vi "Initialization VI.vi"(8 "error in (no error)":errorcluster, 10 "Custom XML":string, 11 "Device Item Ref in":T1 format="%.0x") -> (0 "error out":errorcluster, 3 "Device Item Ref out":T1 format="%.0x")   [LabVIEW 2019, in "FPGA Addon System Explorer.lvlib"]
uses:
  FPGA Addon System Explorer.lvlib
  <vilib>/NI/NI VeriStand Custom Device Import and Export Tool/ImportExport.lvlib
  Addon Shared/FPGA Addon Shared.lvlib
  <vilib>/NI VeriStand/Custom Device API/Custom Device Item Ref.ctl
  <vilib>/NI VeriStand/Custom Device API/Custom Device API.lvlib
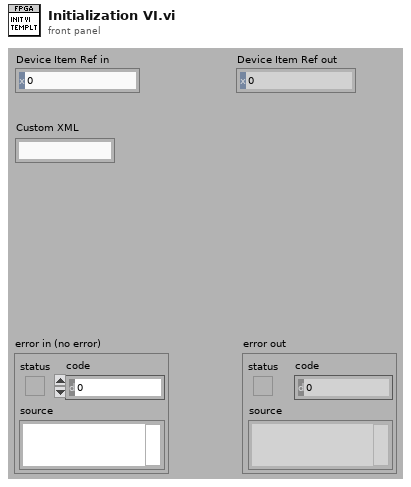
[diagram p1: front panel]
types:
  T1 = typedef "Custom Device API.lvlib/Custom Device Item Ref.ctl" = u64
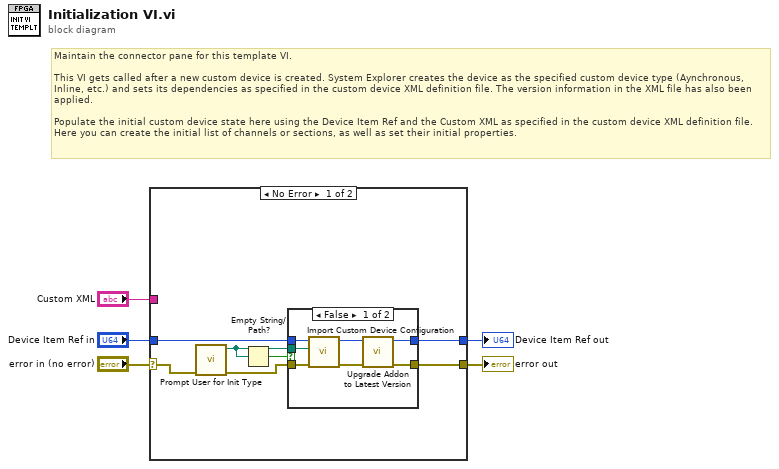
[diagram p0: block diagram]
diagram:
  # "Maintain the connector pane for this template VI.\n\nThis VI gets called after a new custom device is created. System Explorer creates the device as the specified custom device type (Aynchronous, Inline, etc.) and sets its dependencies as specified in the custom device XML definition file. The version information in the XML file has also been applied.\n\nPopulate the initial custom device state here using the Device Item Ref and the Custom XML as specified in the custom device XML definition file. Here you can create the initial list of channels or sections, as well as set their initial properties."
  n1 = case shown="No Error" "error in (no error)" {
    selector: "error in (no error)" -> [w12 w23]
    tunnel: [w9 w23] -> w5
    tunnel: [w7 w22] -> w3
    tunnel: "Device Item Ref in" -> [w6 w22]
    tunnel: "Custom XML" -> [_ _]
    frame No Error {
      n2 = call "Prompt User for Init Type.vi"("error in (no error)"=w12) -> ("error out"=w10:errorcluster, "Path out"=w8:path)  [unwired: 9 in]
      n3 = Empty String/Path?(string/path=w8) -> (empty?=w11:bool)
      n4 = case shown="False" w11 {
        tunnel: w10 -> [w17 w21]
        tunnel: [w16 w21] -> w9
        tunnel: w8 -> [w15 _]
        tunnel: w6 -> [w14 w20]
        tunnel: [w13 w20] -> w7
        frame False {
          n5 = call <vilib>:"Import Custom Device Configuration.vi"("error in (no error)"=w17, "Path"=w15, "NodeID"=w14) -> ("error out"=w19:errorcluster, "NodeID out"=w18:u64)  [unwired: 6 in, 1 out]
          n6 = call "Upgrade Addon to Latest Version.vi"("error in (no error)"=w19, "Device Item Ref in in"=w18) -> ("error out"=w16:errorcluster, "Device Item Ref out"=w13:T1)  [unwired: 8 in]
        }
        frame True {
        }
      }
    }
    frame Error {
    }
  }
  "error out" <- w5
  "Device Item Ref out" <- w3
